vi "Motor_generatespeed.vi"(2 "error in (no error)":errorcluster, 3 "Conversion\n (steps/mm)":dbl[](array[numeric])=[12500.0, 31496.063, 31496.063] format="%#_13g", 4 "Speed (mm/s)":dbl[](array[numeric]) format="%#_13g", 5 "reference":refnum<k7>) -> (0 "error out":errorcluster, 1 "reference out":refnum<k7>)   [LabVIEW 2015]
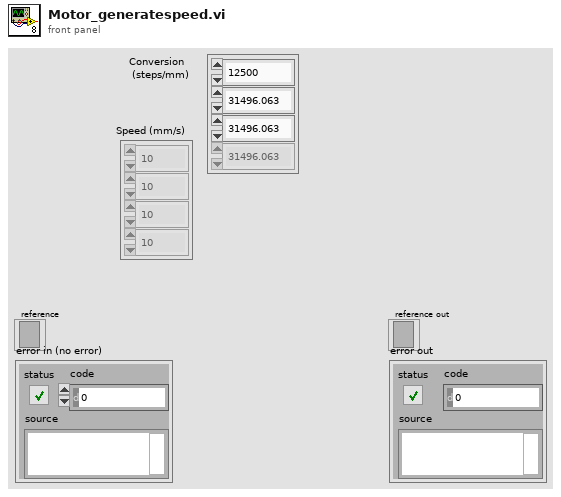
[diagram p1: front panel]
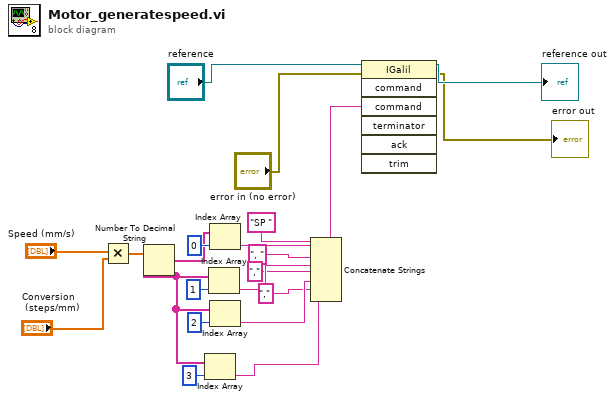
[diagram p0: block diagram]
diagram:
  n1 = Multiply(x="Speed (mm/s)", y="Conversion\n (steps/mm)") -> (x*y=w10:dbl[])
  n2 = Number To Decimal String(number=w10) -> (decimal integer string=w3:string[])  [unwired: 1 in]
  n3 = Index Array(array=w3, index=3) -> (element=w1:string)
  n4 = Index Array(array=w3, index=1) -> (element=w17:string)
  n5 = Index Array(array=w3, index=0) -> (element=w19:string)
  n6 = Index Array(array=w3, index=2) -> (element=w13:string)
  n7 = Concatenate Strings("SP " ("string"), w19, ", " ("string"), w17, "," ("string"), w13, "," ("string"), w1) -> (w5:string)
  n8 = invoke class="IGalil" method="command"(reference="reference", error in="error in (no error)", "command"=w5) -> (reference out=→"reference out":refnum<k7>, error out=→"error out":errorcluster)  [unwired: 4 in, 5 out]
